vi "Constructor.vi"(8 "error in (no error)":errorcluster, 11 "FrozenClams in":refnum<class "FrozenClams.lvclass">) -> (0 "error out":errorcluster, 2 "Ingredients":string, 3 "FrozenClams out":refnum<class "FrozenClams.lvclass">)   [LabVIEW 2013, in "FrozenClams.lvclass"]
uses:
  FrozenClams.lvclass
panel:
  # "§Ú¬O§N­áµð¸Ä"
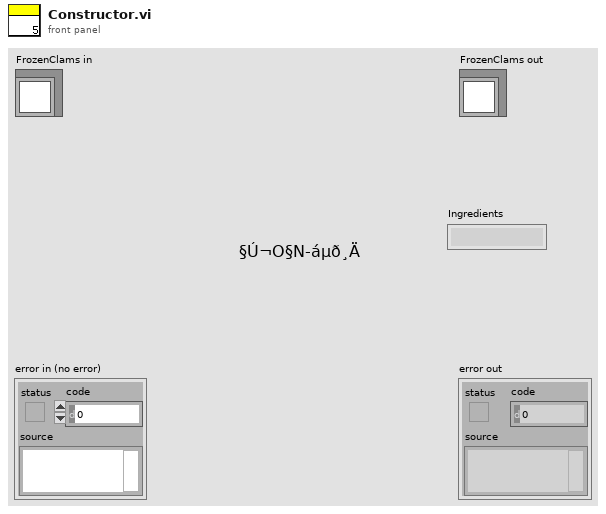
[diagram p1: front panel]
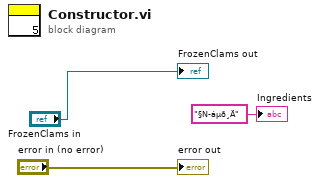
[diagram p0: block diagram]
diagram:
  "error out" <- "error in (no error)"
  "FrozenClams out" <- "FrozenClams in"
  "Ingredients" <- "§N­áµð¸Ä" ("Ingredients")
